vi "SignalMeasurements.vi"(1 "Waveform":waveform(dbl), 4 "error in":errorcluster) -> (14 "magnitude":dbl[](graph), 15 "df":dbl, 16 "f0":dbl, 17 "signal power":dbl, 18 "max frequency":dbl, 19 "error out":errorcluster)   [LabVIEW 2025]
uses:
  <vilib>/express/express analysis/Spectral/Block/exnSpectralBlock spectral measurements peak poly.vi
  <vilib>/express/express analysis/Spectral/Block/exnSpectralBlock spectral measurements peak WFM.vi
  <vilib>/express/express analysis/Spectral/XNode/ExpressSpectralMeasurementsBlockNode.xnode
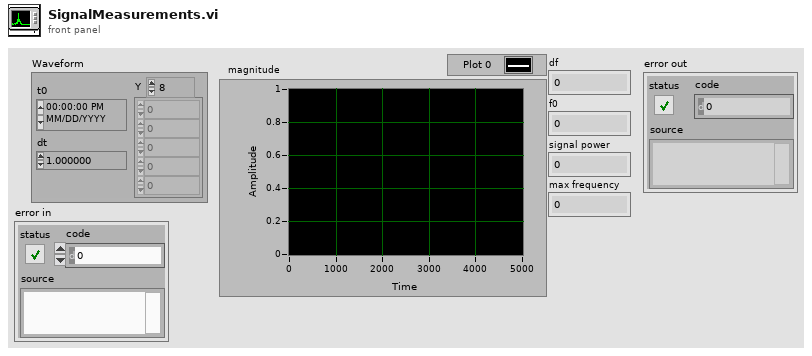
[diagram p1: front panel]
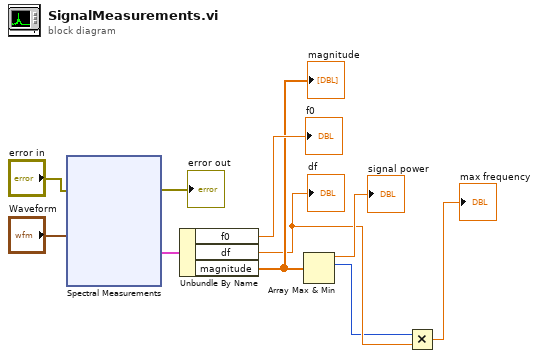
[diagram p0: block diagram]
diagram:
  n1 = xnode "Spectral Measurements"("Signals"="Waveform", "error in (no error)"="error in") -> ("FFT - (Peak)"=w9:cluster{"f0":dbl, "df":dbl, "magnitude":dbl[]}, "error out"=→"error out":errorcluster)  [unwired: 1 out]
  n2 = Unbundle By Name(w9) -> ("f0"=→"f0":dbl, "df"=w5:dbl, "magnitude"=w7:dbl[])
  "magnitude" <- w7
  "df" <- w5
  n3 = Array Max & Min(array=w7) -> (max value=→"signal power":dbl, max index (indices)=w1:i32)  [unwired: 2 out]
  n4 = Multiply(x=w1, y=w5) -> (x*y=→"max frequency":dbl)
